vi "Set MB session in.vi"(10 "MB Serial Master:MB_Master":refnum<class "MB_Master.lvclass">, 11 "DAM0200-Relay in":refnum<class "DAM0200-Relay.lvclass">) -> (3 "DAM0200-Relay out":refnum<class "DAM0200-Relay.lvclass">)   [LabVIEW 2016, in "DAM0200-Relay.lvlib" / "DAM0200-Relay.lvclass"]
uses:
  DAM0200-Relay.lvclass
  <vilib>/Plasmionique/MB Master/MB_Master/MB_Master.lvclass
  DAM0200-Relay.lvclass/DAM0200-Relay.ctl
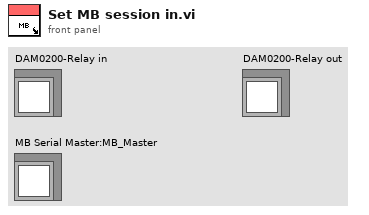
[diagram p1: front panel]
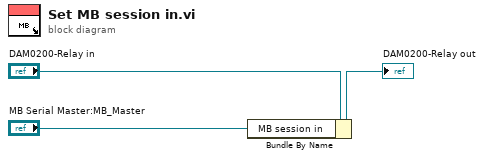
[diagram p0: block diagram]
diagram:
  n1 = Bundle By Name(cluster="DAM0200-Relay in", "MB session in"="MB Serial Master:MB_Master") -> (→"DAM0200-Relay out":refnum<class "DAM0200-Relay.lvclass">)
